vi "FPGA Main - 9035.vi"() -> ()   [LabVIEW 2017]
uses:
  Controls/Logging Settings FPGA.ctl
  Controls/Manual Control FPGA.ctl
  <vilib>/rvi/eio/common/nirviEmuTemplateMethod_errors.vi
  <vilib>/rvi/Emulation/niFpgaGetClockAttributes.vi
  <vilib>/rvi/Emulation/niFpgaSctlEmulationGetInTimedLoop.vi
  <vilib>/rvi/Emulation/niFpgaEmulationReportErrorSimple.vi
  <vilib>/rvi/Emulation/niFpgaProcessEmulError.vi
  <vilib>/rvi/interface/RandomDataEmulation/niFpgaRandomDataHandleErrors.vi
  <vilib>/rvi/Emulation/niFpgaCriticalErrorInLSC.vi
  <vilib>/eio/EIONode/EIONode.xnode
  <vilib>/rvi/DataTransferAndStorage/Container/XNode/niFpgaContainer.xnode
  <vilib>/rvi/interface/RandomDataEmulation/nirviRandomDataFpgaReadWriteTemplate.vi
panel:
  in  "Emergency Shutdown Channel":T1(ring)
  out "Emergency Triggered":bool
  in  "Emergency Normally Open/Closed":bool
  in  "Actuator Settings":T2 {"Emergency State" items=["Closed", "Open"]; "Output Port" items=["DIDO/DO0", "DIDO/DO1", "DIDO/DO2", "DIDO/DO3", "DIDO/DO4", "DIDO/DO5", "DIDO/DO6", "DIDO/DO7", "DIDO/DO8", "DIDO/DO9", "DIDO/DO10", "DIDO/DO11", "DIDO/DO12", "DIDO/DO13", "DIDO/DO14", "DIDO/DO15", "PWM/DO0", "PWM/DO1", "PWM/DO2", "PWM/DO3", "PWM/DO4", "PWM/DO5", "PWM/DO6", "PWM/DO7"]; "Unpowered State" items=["Closed", "Opened"]}
  in  "Logging Settings [Ticks]":T3
  out "LC FIFO Timed Out":bool
  out "PS FIFO Timed Out":bool
  in  "Poll Rate [Ticks]":u32
  in  "Logging?":bool
  out "TC FIFO Timed Out":bool
  in  "High Speed?":bool
  out "Automated Sequence Timer":i32
  in  "Emergency Shutdown":bool
  in  "Start Automated Sequence":bool
  in  "Manual Mode":bool=TRUE
  out "FPGA States":T4(ring)
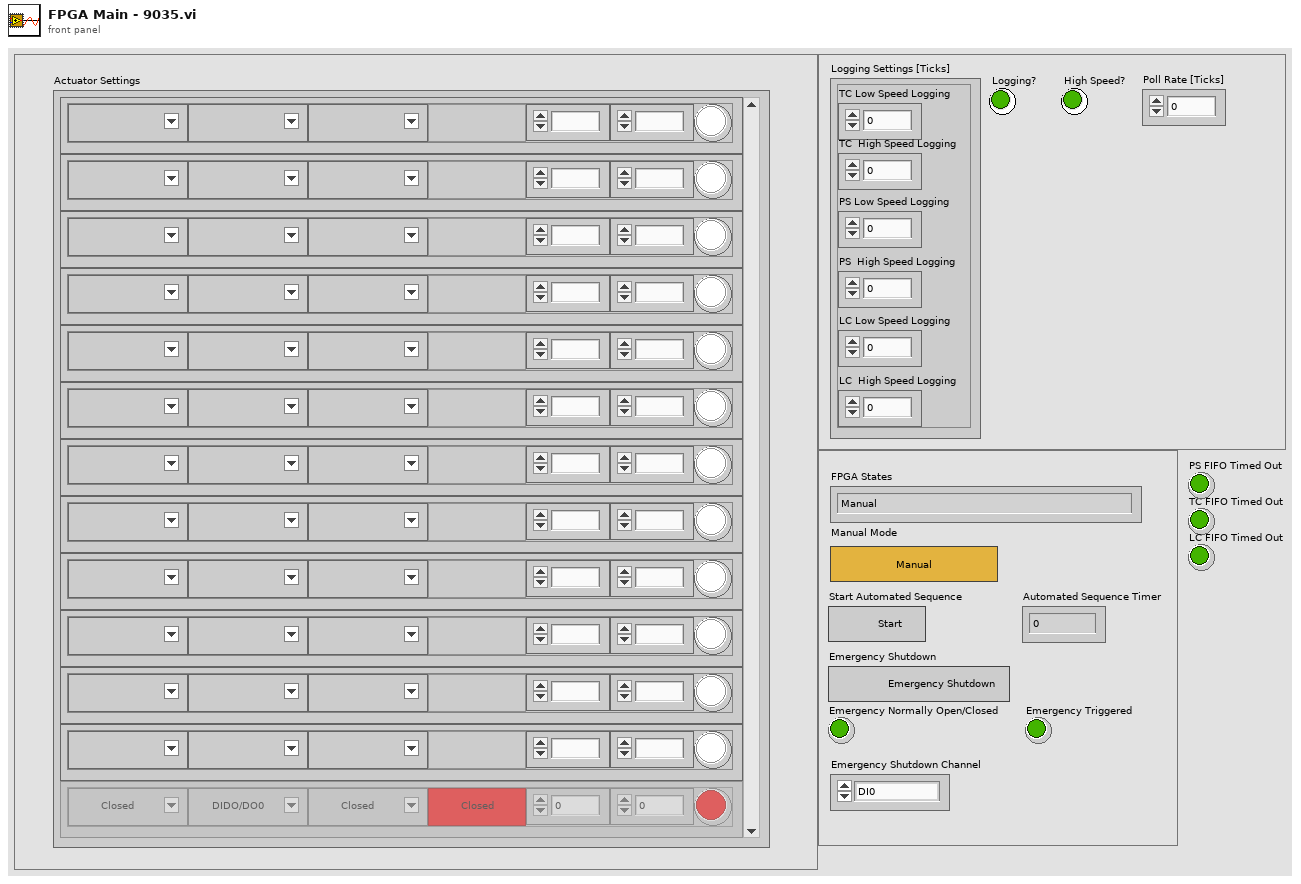
[diagram p1: front panel]
types:
  T1 = enum16{"DI0", "DI1", "DI2", "DI3", "DI4", "DI5", "DI7", "DI6", "DI8", "DI9", "DI10", "DI11", "DI12", "DI13", "DI14", "DI15"}
  T2 = typedef "Manual Control FPGA.ctl" = cluster{"Unpowered State":u8, "Output Port":u8, "Emergency State":u8, "Blank Button":bool, "Open Time [ms]":fxp<+/-,18,18>, "Close Time [ms]":fxp<+/-,18,18>, "Active":bool}[]
  T3 = typedef "Logging Settings FPGA.ctl" = cluster{"TC Low Speed Logging":u32, "TC  High Speed Logging":u32, "PS Low Speed Logging":u32, "PS  High Speed Logging":u32, "LC Low Speed Logging":u32, "LC  High Speed Logging":u32}
  T4 = enum16{"Manual", "Standby", "Automated Sequence", "Automated Sequence End", "Emergency"}
  T5 = cluster{"Unpowered State":u8, "Output Port":u8, "Emergency State":u8, "Blank Button":bool, "Open Time [ms]":fxp<+/-,18,18>, "Close Time [ms]":fxp<+/-,18,18>, "Active":bool}
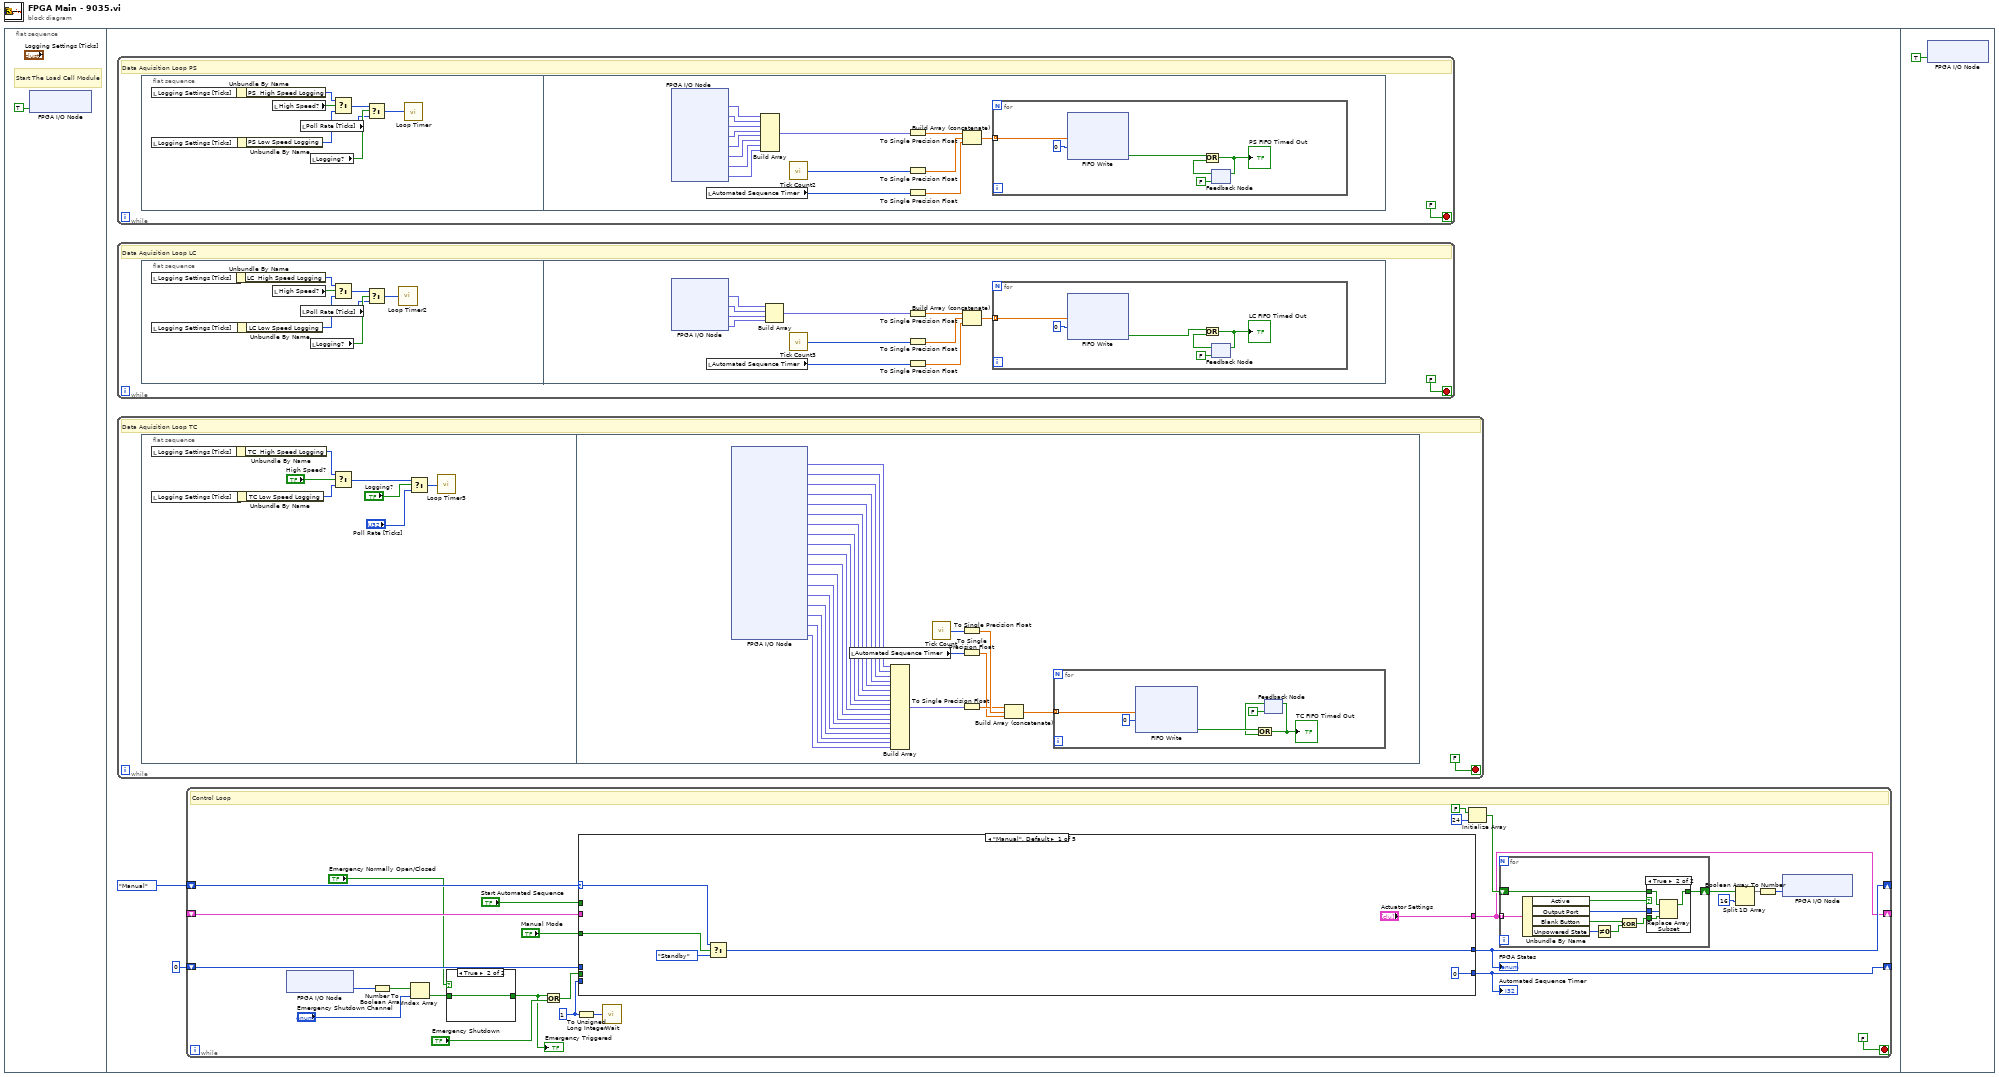
[diagram p0: block diagram]
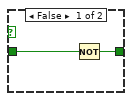
[diagram p2: hidden frame]
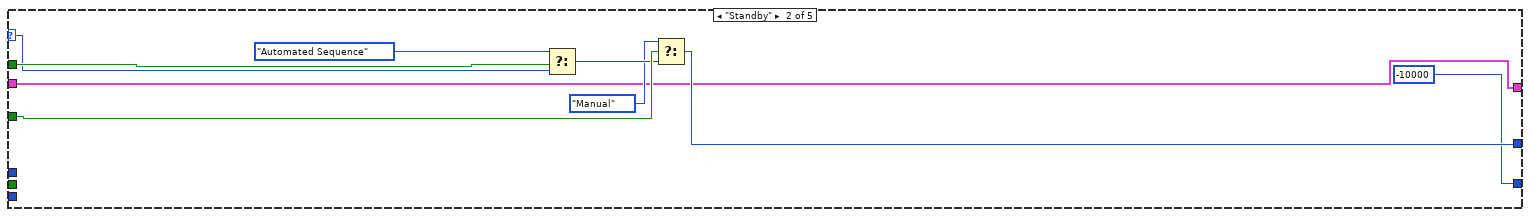
[diagram p4: hidden frame]
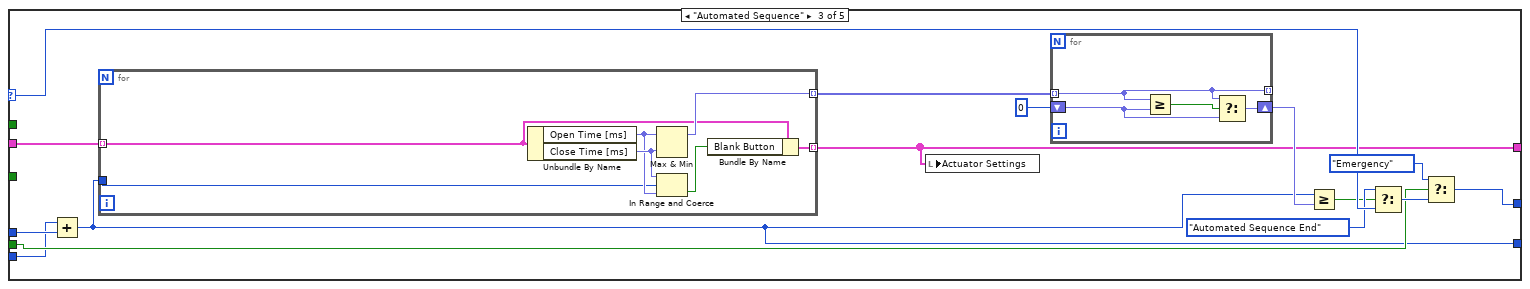
[diagram p5: hidden frame]
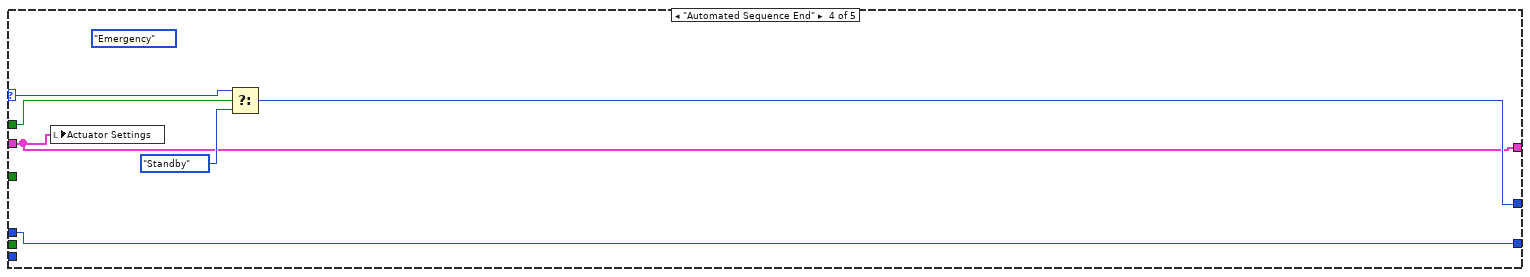
[diagram p6: hidden frame]
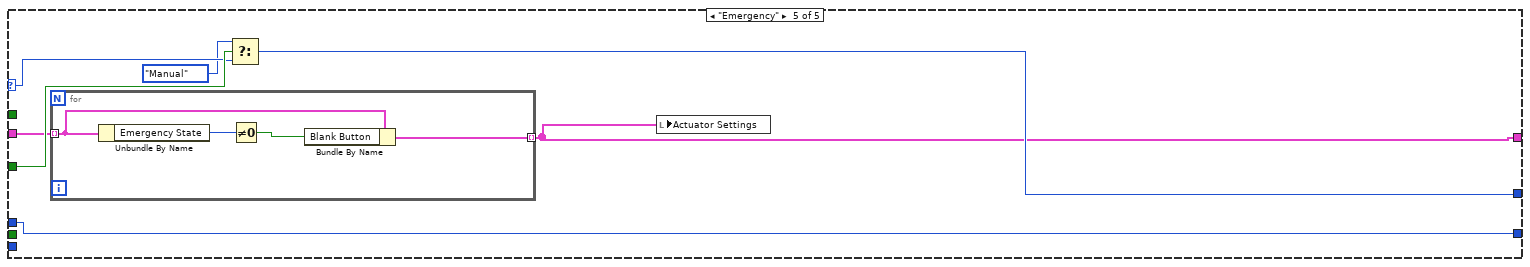
[diagram p7: hidden frame]
diagram:
  n1 = flat-sequence {
    frame #0 {
      # "Start The Load Cell Module"
      n2 = xnode "FPGA I/O Node"("Mod2/Start"=TRUE ("LC/Start")) -> ()  [unwired: 1 in, 1 out]
    }
    frame #1 {
      n3 = while {
        stop <- FALSE stop-if-true
        # "Data Aquisition Loop PS"
        n4 = flat-sequence {
          frame #0 {
            n5 = local read "Logging Settings [Ticks]"() -> (w140:T3)
            n6 = local read "Logging Settings [Ticks]"() -> (w138:T3)
            n7 = Unbundle By Name(w140) -> ("PS  High Speed Logging"=w135:u32)
            n8 = Unbundle By Name(w138) -> ("PS Low Speed Logging"=w134:u32)
            n9 = local read "High Speed?"() -> (w139:bool)
            n10 = local read "Poll Rate [Ticks]"() -> (w136:u32)
            n11 = local read "Logging?"() -> (w137:bool)
            n12 = Select(t=w135, s=w139, f=w134) -> (s? t:f=w141:u32)
            n13 = Select(t=w141, s=w137, f=w136) -> (s? t:f=w133:u32)
            n14 = call "Loop Timer"("Count(Ticks)"=w133) -> ()  [unwired: 1 out]
          }
          frame #1 {
            n15 = xnode "FPGA I/O Node"() -> ("Mod4/AI0"=w156:fxp<+/-,21,-4>, "Mod4/AI1"=w150:fxp<+/-,21,-4>, "Mod4/AI2"=w149:fxp<+/-,21,-4>, "Mod4/AI3"=w148:fxp<+/-,21,-4>, "Mod4/AI4"=w147:fxp<+/-,21,-4>, "Mod4/AI5"=w146:fxp<+/-,21,-4>, "Mod4/AI6"=w145:fxp<+/-,21,-4>, "Mod4/AI7"=w144:fxp<+/-,21,-4>)  [unwired: 8 in, 8 out]
            n16 = local read "Automated Sequence Timer"() -> (w143:i32)
            n17 = Build Array(w156, w150, w149, w148, w147, w146, w145, w144) -> (w155:fxp<+/-,21,-4>[])
            n18 = call "Tick Count2"() -> ("Tick Count(uSec)"=w153:u32)
            n19 = To Single Precision Float(number=w155) -> (single precision float=w151:sgl[])
            n20 = To Single Precision Float(number=w153) -> (single precision float=w152:sgl)
            n21 = To Single Precision Float(number=w143) -> (single precision float=w142:sgl)
            n22 = Build Array (concatenate)(w151, w152, w142) -> (w154:sgl[])
            n23 = for {
              tunnel: w154 -> [w162] mode=indexing
              n24 = xnode ("FIFO Write")("Element"=w162, "Timeout"=0) -> ("Timed Out?"=w160:bool)  [unwired: 1 in, 1 out]
              n25 = feedback #1(FALSE ("Timed Out?")) -> (w157:bool)
              n26 = Or(x=w160, y=w157) -> (x .or. y?=w158:bool)
              "PS FIFO Timed Out" <- w158
              n27 = feedback-in #1(w158) -> ()
            }
          }
        }
      }
      n28 = while {
        stop <- FALSE stop-if-true
        # "Data Aquisition Loop LC"
        n29 = flat-sequence {
          frame #0 {
            n30 = local read "Logging Settings [Ticks]"() -> (w114:T3)
            n31 = local read "Logging Settings [Ticks]"() -> (w112:T3)
            n32 = Unbundle By Name(w114) -> ("LC  High Speed Logging"=w108:u32)
            n33 = Unbundle By Name(w112) -> ("LC Low Speed Logging"=w109:u32)
            n34 = local read "High Speed?"() -> (w113:bool)
            n35 = local read "Poll Rate [Ticks]"() -> (w110:u32)
            n36 = local read "Logging?"() -> (w111:bool)
            n37 = Select(t=w108, s=w113, f=w109) -> (s? t:f=w107:u32)
            n38 = Select(t=w107, s=w111, f=w110) -> (s? t:f=w106:u32)
            n39 = call "Loop Timer2"("Count(Ticks)"=w106) -> ()  [unwired: 1 out]
          }
          frame #1 {
            n40 = xnode "FPGA I/O Node"() -> ("Mod2/AI0"=w125:fxp<+/-,24,-4>, "Mod2/AI1"=w119:fxp<+/-,24,-4>, "Mod2/AI2"=w118:fxp<+/-,24,-4>, "Mod2/AI3"=w117:fxp<+/-,24,-4>)  [unwired: 4 in, 4 out]
            n41 = local read "Automated Sequence Timer"() -> (w116:i32)
            n42 = Build Array(w125, w119, w118, w117) -> (w124:fxp<+/-,24,-4>[])
            n43 = call "Tick Count3"() -> ("Tick Count(uSec)"=w122:u32)
            n44 = To Single Precision Float(number=w124) -> (single precision float=w120:sgl[])
            n45 = To Single Precision Float(number=w122) -> (single precision float=w121:sgl)
            n46 = To Single Precision Float(number=w116) -> (single precision float=w115:sgl)
            n47 = Build Array (concatenate)(w120, w121, w115) -> (w123:sgl[])
            n48 = for {
              tunnel: w123 -> [w131] mode=indexing
              n49 = xnode ("FIFO Write")("Element"=w131, "Timeout"=0) -> ("Timed Out?"=w129:bool)  [unwired: 1 in, 1 out]
              n50 = feedback #2(FALSE ("Timed Out?")) -> (w126:bool)
              n51 = Or(x=w129, y=w126) -> (x .or. y?=w127:bool)
              "LC FIFO Timed Out" <- w127
              n52 = feedback-in #2(w127) -> ()
            }
          }
        }
      }
      n53 = while {
        stop <- FALSE stop-if-true
        # "Data Aquisition Loop TC"
        n54 = flat-sequence {
          frame #0 {
            n55 = local read "Logging Settings [Ticks]"() -> (w168:T3)
            n56 = local read "Logging Settings [Ticks]"() -> (w166:T3)
            n57 = Unbundle By Name(w168) -> ("TC  High Speed Logging"=w167:u32)
            n58 = Unbundle By Name(w166) -> ("TC Low Speed Logging"=w165:u32)
            n59 = Select(t=w167, s="High Speed?", f=w165) -> (s? t:f=w170:u32)
            n60 = Select(t=w170, s="Logging?", f="Poll Rate [Ticks]") -> (s? t:f=w164:u32)
            n61 = call "Loop Timer3"("Count(Ticks)"=w164) -> ()  [unwired: 1 out]
          }
          frame #1 {
            n62 = xnode "FPGA I/O Node"() -> ("Mod1/TC0"=w197:fxp<+/-,24,-2>, "Mod1/TC1"=w191:fxp<+/-,24,-2>, "Mod1/TC2"=w190:fxp<+/-,24,-2>, "Mod1/TC3"=w189:fxp<+/-,24,-2>, "Mod1/TC4"=w188:fxp<+/-,24,-2>, "Mod1/TC5"=w187:fxp<+/-,24,-2>, "Mod1/TC6"=w186:fxp<+/-,24,-2>, "Mod1/TC7"=w185:fxp<+/-,24,-2>, "Mod1/TC8"=w184:fxp<+/-,24,-2>, "Mod1/TC9"=w183:fxp<+/-,24,-2>, "Mod1/TC10"=w182:fxp<+/-,24,-2>, "Mod1/TC11"=w181:fxp<+/-,24,-2>, "Mod1/TC12"=w180:fxp<+/-,24,-2>, "Mod1/TC13"=w179:fxp<+/-,24,-2>, "Mod1/TC14"=w178:fxp<+/-,24,-2>, "Mod1/TC15"=w177:fxp<+/-,24,-2>, "Mod1/Autozero"=w176:fxp<+/-,24,-2>, "Mod1/CJC"=w175:fxp<+/-,24,-2>)  [unwired: 18 in, 18 out]
            n63 = local read "Automated Sequence Timer"() -> (w174:i32)
            n64 = Build Array(w197, w191, w190, w189, w188, w187, w186, w185, w184, w183, w182, w181, w180, w179, w178, w177, w176, w175) -> (w196:fxp<+/-,24,-2>[])
            n65 = call "Tick Count"() -> ("Tick Count(uSec)"=w194:u32)
            n66 = To Single Precision Float(number=w194) -> (single precision float=w193:sgl)
            n67 = To Single Precision Float(number=w174) -> (single precision float=w173:sgl)
            n68 = To Single Precision Float(number=w196) -> (single precision float=w192:sgl[])
            n69 = Build Array (concatenate)(w192, w193, w173) -> (w195:sgl[])
            n70 = for {
              tunnel: w195 -> [w203] mode=indexing
              n71 = xnode ("FIFO Write")("Element"=w203, "Timeout"=0) -> ("Timed Out?"=w201:bool)  [unwired: 1 in, 1 out]
              n72 = feedback #3(FALSE ("Timed Out?")) -> (w198:bool)
              n73 = Or(x=w201, y=w198) -> (x .or. y?=w199:bool)
              "TC FIFO Timed Out" <- w199
              n74 = feedback-in #3(w199) -> ()
            }
          }
        }
      }
      n75 = while {
        shift-right: [w28] -> _
        shift-left: T4."Manual" ("FPGA States") -> [w29]
        shift-right: [w11] -> _
        shift-left: _ -> [w19]
        shift-right: [w24] -> _
        shift-left: 0 -> [w23]
        stop <- FALSE stop-if-true
        w22 = 1 ("Count(mSec)")
        # "Control Loop"
        n76 = xnode "FPGA I/O Node"() -> ("Mod3/DI15:0"=w4:u16)  [unwired: 1 in, 1 out]
        n77 = Number To Boolean Array(number=w4) -> (Boolean array=w5:bool[])
        n78 = Index Array(array=w5, index="Emergency Shutdown Channel") -> (element=w6:bool)
        n79 = case shown="True" "Emergency Normally Open/Closed" {
          tunnel: w6 -> [w31 w32]
          tunnel: [w30 w32] -> w9
          frame False {
            n80 = Not(x=w31) -> (.not. x?=w30:bool)
          }
          frame True {
          }
        }
        "Emergency Triggered" <- w9
        n81 = Or(x=w9, y="Emergency Shutdown") -> (x .or. y?=w10:bool)
        n82 = To Unsigned Long Integer(number=w22) -> (unsigned 32bit integer=w21:u32)
        n83 = case shown="\"Manual\", Default" w29 {
          selector: w29 -> [w52 w60 w74 w91 w98]
          tunnel: [w49 w55 w75 w89 w96] -> w28
          tunnel: w10 -> [_ _ w71 _ _]
          tunnel: "Start Automated Sequence" -> [_ w61 _ w92 _]
          tunnel: "Manual Mode" -> [w50 w58 _ _ w99]
          tunnel: [0 -10000 w64 w93 w100] -> w24
          tunnel: w23 -> [_ _ w70 w93 w100]
          tunnel: w22 -> [_ _ w69 _ _]
          tunnel: ["Actuator Settings" w53 w63 w88 w94] -> w11
          tunnel: w19 -> [_ w53 w65 w88 w95]
          frame "Manual", Default {
            n84 = Select(t=w52, s=w50, f=T4."Standby") -> (s? t:f=w49:T4)
          }
          frame "Standby" {
            n85 = Select(t=T4."Automated Sequence", s=w61, f=w60) -> (s? t:f=w57:T4)
            n86 = Select(t=T4."Manual", s=w58, f=w57) -> (s? t:f=w55:T4)
          }
          frame "Automated Sequence" {
            n87 = Add(x=w69, y=w70) -> (x+y=w64:i32)
            n88 = for {
              tunnel: w65 -> [w79] mode=indexing
              tunnel: [w83] -> w66 mode=indexing
              tunnel: w64 -> [w77]
              tunnel: [w78] -> w63 mode=indexing
              n89 = Unbundle By Name(w79) -> ("Open Time [ms]"=w81:fxp<+/-,18,18>, "Close Time [ms]"=w82:fxp<+/-,18,18>)
              n90 = Max & Min(x=w81, y=w82) -> (max(x,y)=w83:fxp<+/-,18,18>)  [unwired: 1 out]
              n91 = In Range and Coerce(upper limit=w82, x=w77, lower limit=w81) -> (In Range?=w80:bool)  [unwired: 1 out]
              n92 = Bundle By Name(cluster=w79, "Blank Button"=w80) -> (w78:T5)
            }
            n93 = local write "Actuator Settings"(w63) -> ()
            n94 = for {
              tunnel: [w84] -> _ mode=indexing
              shift-right: [w87] -> w67
              shift-left: 0 ("y") -> [w85]
              tunnel: w66 -> [w84] mode=indexing
              n95 = Greater Or Equal?(x=w84, y=w85) -> (x >= y?=w86:bool)
              n96 = Select(t=w84, s=w86, f=w85) -> (s? t:f=w87:fxp<+/-,32,32>)
            }
            n97 = Greater Or Equal?(x=w64, y=w67) -> (x >= y?=w62:bool)
            n98 = Select(t=T4."Automated Sequence End", s=w62, f=w74) -> (s? t:f=w72:T4)
            n99 = Select(t=T4."Emergency", s=w71, f=w72) -> (s? t:f=w75:T4)
          }
          frame "Automated Sequence End" {
            (unwired) T4."Emergency" ("t")
            n100 = local write "Actuator Settings"(w88) -> ()
            n101 = Select(t=w91, s=w92, f=T4."Standby" ("FPGA States")) -> (s? t:f=w89:T4)
          }
          frame "Emergency" {
            n102 = for {
              tunnel: w95 -> [w104] mode=indexing
              tunnel: [w101] -> w94 mode=indexing
              n103 = Unbundle By Name(w104) -> ("Emergency State"=w102:u8)
              n104 = Not Equal To 0?(x=w102) -> (x != 0?=w103:bool)
              n105 = Bundle By Name(cluster=w104, "Blank Button"=w103) -> (w101:T5)
            }
            n106 = Select(t=T4."Manual", s=w99, f=w98) -> (s? t:f=w96:T4)
            n107 = local write "Actuator Settings"(w94) -> ()
          }
        }
        "FPGA States" <- w28
        "Automated Sequence Timer" <- w24
        n108 = call "Wait"("Count(mSec)"=w21) -> ()  [unwired: 1 out]
        n109 = Initialize Array(FALSE, 24 ("dimension size")) -> (w17:bool[])
        n110 = for {
          tunnel: w11 -> [w41] mode=indexing
          shift-right: [w36] -> w16
          shift-left: w17 -> [w37]
          n111 = Unbundle By Name(w41) -> ("Active"=w33:bool, "Output Port"=w35:u8, "Blank Button"=w40:bool, "Unpowered State"=w39:u8)
          n112 = Not Equal To 0?(x=w39) -> (x != 0?=w38:bool)
          n113 = Exclusive Or(1:w38, 2:w40) -> (0:w34:bool)
          n114 = case shown="True" w33 {
            tunnel: w37 -> [w42 w46]
            tunnel: [w42 w45] -> w36
            tunnel: w35 -> [_ w44]
            tunnel: w34 -> [_ w43]
            frame False {
            }
            frame True {
              n115 = Replace Array Subset(array=w46, new element=w43, index=w44) -> (w45:bool[])
            }
          }
        }
        n116 = Split 1D Array(array=w16, index=16) -> (first subarray=w13:bool[])  [unwired: 1 out]
        n117 = Boolean Array To Number(Boolean array=w13) -> (number=w14:u16)
        n118 = xnode "FPGA I/O Node"("Mod3/DO15:0"=w14) -> ()  [unwired: 1 in, 1 out]
      }
    }
    frame #2 {
      n119 = xnode "FPGA I/O Node"("Mod2/Stop"=TRUE ("LC/Start")) -> ()  [unwired: 1 in, 1 out]
    }
  }
